vi "Practica 5 - Ejercicio Ecuacion.vi"() -> ()   [LabVIEW 2023]
panel:
  out "Y2":dbl
  out "Y1":dbl
  in  "c":dbl
  in  "m":dbl
  in  "x":dbl
  in  "E":dbl
  in  "D":dbl
  in  "C":dbl
  in  "B":dbl
  in  "A":dbl
  # "Ecuaciones Propuetas"
  # "( A   B   C  )+(   D   E   )  ="
  # "(  x  m  ) + c ="
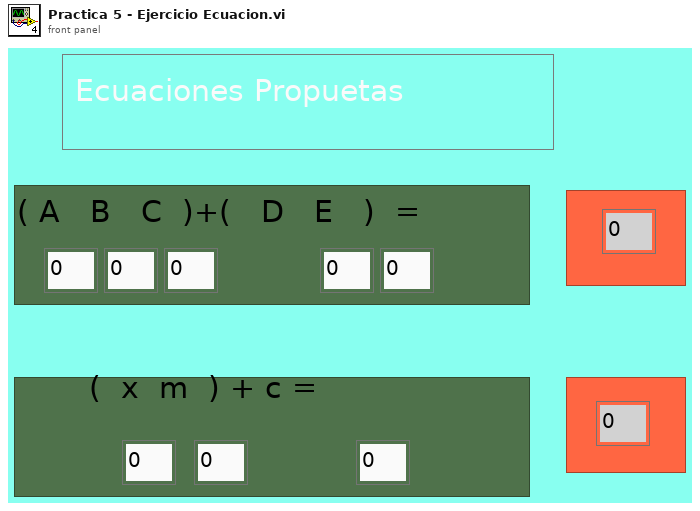
[diagram p1: front panel]
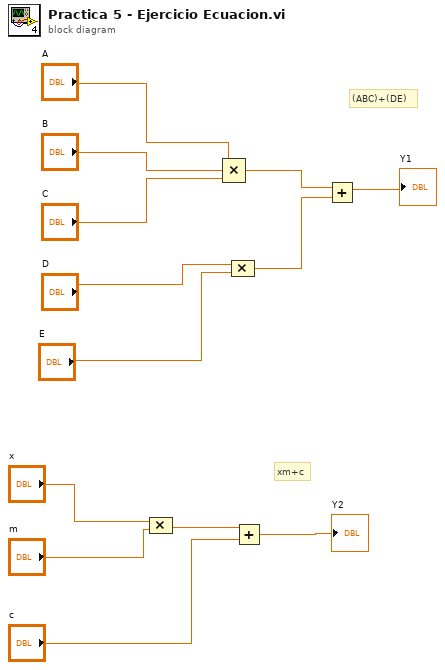
[diagram p0: block diagram]
diagram:
  # "xm+c"
  # "(ABC)+(DE)"
  n1 = Compound Arithmetic op=MULTIPLY("x", "m") -> (w3:dbl)
  n2 = Compound Arithmetic op=MULTIPLY("A", "B", "C") -> (w7:dbl)
  n3 = Compound Arithmetic op=MULTIPLY("D", "E") -> (w8:dbl)
  n4 = Add(x=w3, y="c") -> (x+y=→"Y2":dbl)
  n5 = Add(x=w7, y=w8) -> (x+y=→"Y1":dbl)
